vi "CODCr参数WR (子VI) .vi"(0 "STEP":enum16{"read", "writekb", "写入消解温度时间"}(ring)=enum."writekb", 1 "曲线斜率K":sgl, 2 "曲线斜率B":sgl, 3 "消解温度":u16, 4 "消解时长":u16, 5 "Error in":errorcluster caption="Error in (no error)") -> (14 "关键参数区":T1, 19 "error out":errorcluster)   [LabVIEW 2016]
uses:
  <vilib>/Plasmionique/MB Master/MB Master.lvlib
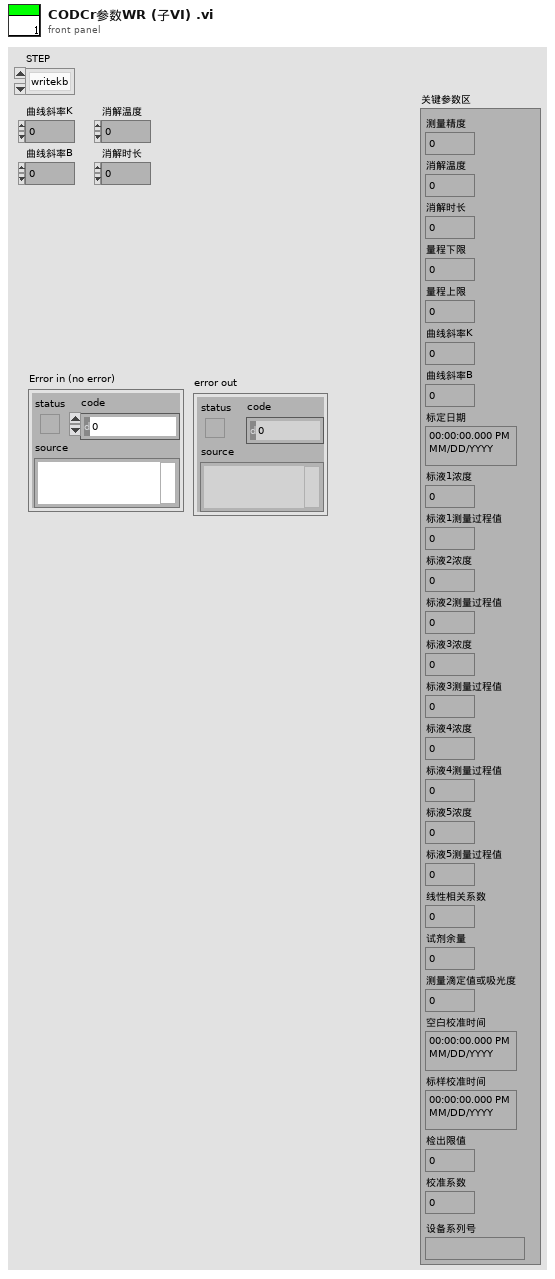
[diagram p1: front panel]
types:
  T1 = cluster{"测量精度":u16, "消解温度":u16, "消解时长":u16, "量程下限":sgl, "量程上限":sgl, "曲线斜率K":sgl, "曲线斜率B":sgl, "标定日期":timestamp, "标液1浓度":sgl, "标液1测量过程值":sgl, "标液2浓度":sgl, "标液2测量过程值":sgl, "标液3浓度":sgl, "标液3测量过程值":sgl, "标液4浓度":sgl, "标液4测量过程值":sgl, "标液5浓度":sgl, "标液5测量过程值":sgl, "线性相关系数":sgl, "试剂余量":u32, "测量滴定值或吸光度":sgl, "空白校准时间":timestamp, "标样校准时间":timestamp, "检出限值":sgl, "校准系数":sgl, "设备系列号":string}
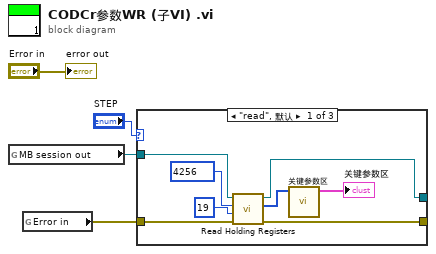
[diagram p0: block diagram]
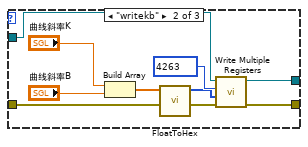
[diagram p2: hidden frame]
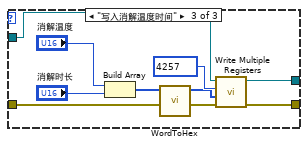
[diagram p3: hidden frame]
diagram:
  n1 = global read "CODcr全局变量.vi" "MB session out"() -> (w1:refnum<class "MB_Master.lvclass">)
  n2 = global read "CODcr全局变量.vi" "Error in"() -> (w3:errorcluster)
  n3 = case shown="\"read\", 默认" "STEP" {
    tunnel: w1 -> [w12 w18 w30]
    tunnel: w3 -> [w11 w17 w29]
    tunnel: [w6 w14 w28] -> _
    tunnel: [w5 w13 w27] -> _
    frame "read", Default {
      n4 = call <vilib>:"Read Holding Registers.vi"("error in (no error)"=w11, "quantity"=u16 19 ("number of holding registers"), "starting address"=u16 4256, "MB session in"=w12) -> ("error out"=w5:errorcluster, "Registers"=w8:u16[], "MB session out"=w6:refnum<class "MB_Master.lvclass">)  [unwired: 5 in]
      n5 = call "关键参数区.vi"("数组"=w8) -> ("关键参数区"=→"关键参数区":T1)  [unwired: 10 in]
    }
    frame "writekb" {
      n6 = Build Array("曲线斜率K", "曲线斜率B") -> (w19:sgl[])
      n7 = call "FloatToHex.vi"("浮点数"=w19) -> ("DCBA整形输出"=w15:u16[])  [unwired: 10 in]
      n8 = call <vilib>:"Write Multiple Registers.vi"("error in (no error)"=w17, "values"=w15, "starting address"=u16 4263, "MB session in"=w18) -> ("error out"=w13:errorcluster, "MB session out"=w14:refnum<class "MB_Master.lvclass">)  [unwired: 6 in]
    }
    frame "写入消解温度时间" {
      n9 = Build Array("消解温度", "消解时长") -> (w23:u16[])
      n10 = call "WordToHex.vi"("WORD"=w23) -> ("数组"=w22:u16[])  [unwired: 10 in]
      n11 = call <vilib>:"Write Multiple Registers.vi"("error in (no error)"=w29, "values"=w22, "starting address"=u16 4257, "MB session in"=w30) -> ("error out"=w27:errorcluster, "MB session out"=w28:refnum<class "MB_Master.lvclass">)  [unwired: 6 in]
    }
  }
  "error out" <- "Error in"
